vi "Async Tree Load Finished.vi"(8 "error in (no error)":errorcluster, 10 "error?":errorcluster, 11 "QControlWizard in":refnum<class "QControl Creation Wizard.lvclass">) -> (0 "error out":errorcluster, 3 "QControlWizard out":refnum<class "QControl Creation Wizard.lvclass">)   [LabVIEW 2015, in "QControl Creation Wizard.lvclass"]
uses:
  QControl Creation Wizard.lvclass
  QControl Creation Wizard.lvclass/QControl Creation Wizard.ctl
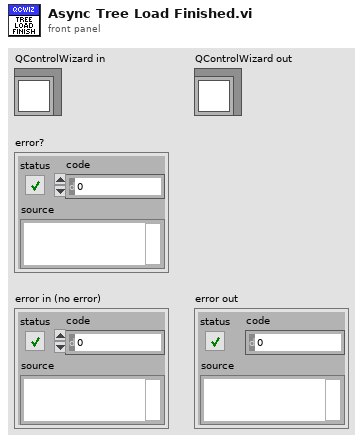
[diagram p1: front panel]
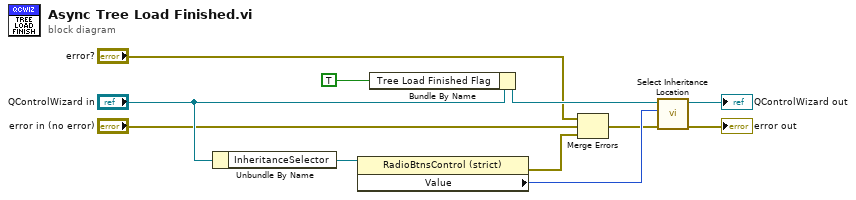
[diagram p0: block diagram]
diagram:
  n1 = Unbundle By Name("QControlWizard in") -> ("InheritanceSelector"=w6:refnum<vi>)
  n2 = property class="RadioBtnsControl (strict)"(reference=w6) -> (error out=w2:errorcluster, "Value"=w9:enum32{"Tree", "Path"})  [unwired: 1 in, 1 out]
  n3 = Bundle By Name(cluster="QControlWizard in", "Tree Load Finished Flag"=TRUE) -> (w5:refnum<class "QControl Creation Wizard.lvclass">)
  n4 = Merge Errors("error?", "error in (no error)", w2) -> (w7:errorcluster)
  n5 = call "Select Inheritance Location.vi"("error in (no error)"=w7, "NewVal"=w9, "QControlWizard in"=w5) -> ("error out"=→"error out":errorcluster, "QControlWizard (dup)"=→"QControlWizard out":refnum<class "QControl Creation Wizard.lvclass">)  [unwired: 7 in]
